vi "lib Create Folder If Necessary.vi"(8 "error in (no error)":errorcluster, 11 "Folder":path) -> (0 "error out":errorcluster, 3 "Folder dup":path)   [LabVIEW 2024]
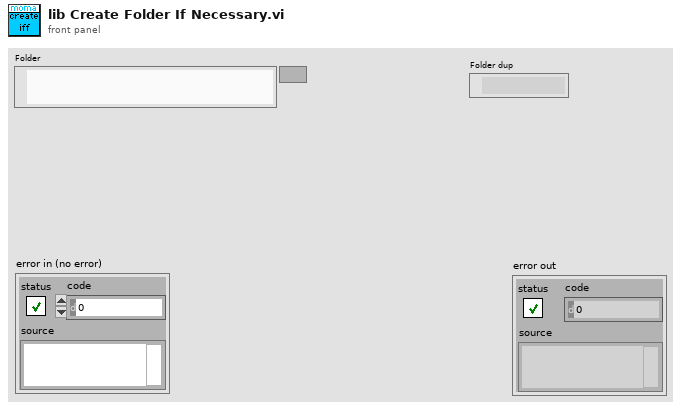
[diagram p1: front panel]
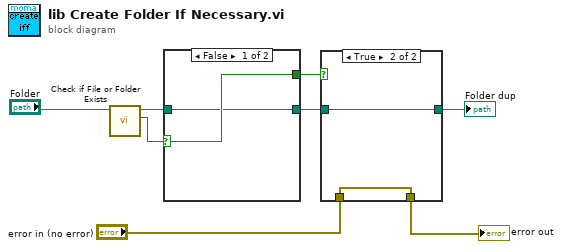
[diagram p0: block diagram]
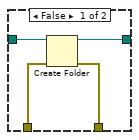
[diagram p2: hidden frame]
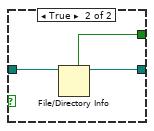
[diagram p3: hidden frame]
diagram:
  n1 = call <vilib>:"Check if File or Folder Exists.vi"("path"="Folder") -> ("file or folder exists?"=w7:bool, "dup path"=w6:path)  [unwired: 8 in, 1 out]
  n2 = case shown="False" w7 {
    selector: w7 -> [w10 _]
    tunnel: w6 -> [w9 w13]
    tunnel: [w10 w12] -> w5
    tunnel: [w9 w11] -> w4
    frame False {
    }
    frame True {
      n3 = File/Directory Info(path=w13) -> (path out=w11:path, directory=w12:bool)  [unwired: 1 in, 5 out]
    }
  }
  n4 = case shown="True" w5 {
    tunnel: w4 -> [w17 w19]
    tunnel: [w16 w19] -> w3
    tunnel: "error in (no error)" -> [w15 w18]
    tunnel: [w14 w18] -> w1
    frame False {
      n5 = Create Folder(path (use dialog)=w17, error in=w15) -> (created path=w16:path, error out=w14:errorcluster)  [unwired: 1 in, 1 out]
    }
    frame True {
    }
  }
  "error out" <- w1
  "Folder dup" <- w3
